vi "Read_Write_Heartbeat_VI.vi"() -> ()   [LabVIEW 2017]
uses:
  b0f9d034-c42f-4ddb-9695-d4b8d01b2041.vi
  <vilib>/Plasmionique/MB Master/MB_Master_TCP/MB_Master_TCP.lvclass
  C:/Program Files (x86)/National Instruments/LabVIEW 2017/vi.lib/Plasmionique/MB Master/MB_Master/MB_Master.lvclass
  <vilib>/Plasmionique/MB Master/MB Master.lvlib
panel:
  out "Heartbeat Value to BMS":i32
  out "BMS IP Address":string
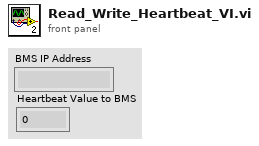
[diagram p1: front panel]
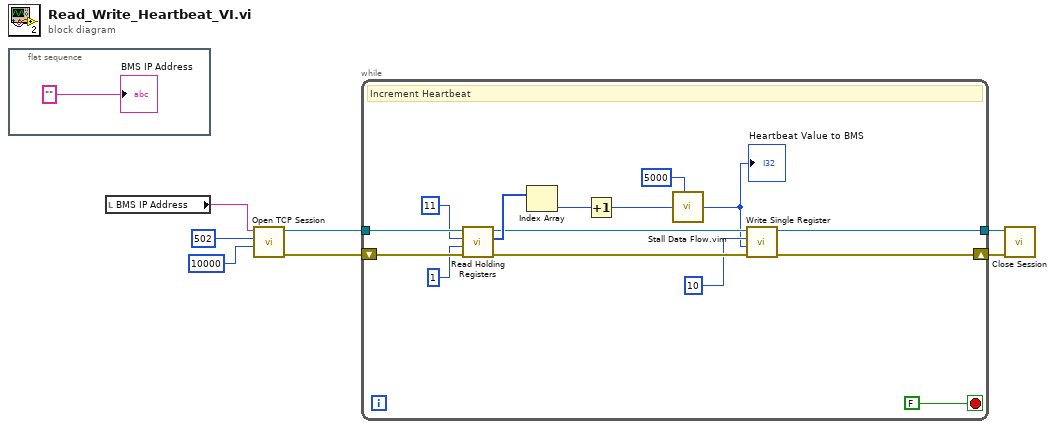
[diagram p0: block diagram]
diagram:
  n1 = flat-sequence {
    frame #0 {
      "BMS IP Address" <- "" ("String")
    }
  }
  n2 = local read "BMS IP Address"() -> (w3:string)
  n3 = call <vilib>:"Open TCP Session.vi"("Timeout (10000)"=10000, "Port (502)"=u16 502, "IP Address"=w3) -> ("error out"=w6:errorcluster, "MB_TCP session"=w7:refnum<class "MB_Master_TCP.lvclass">)  [unwired: 7 in]
  n4 = while {
    tunnel: w7 -> [w22]
    shift-right: [w11] -> w2
    shift-left: w6 -> [w21]
    tunnel: [w10] -> w1
    stop <- FALSE stop-if-true
    # "Increment Heartbeat"
    n5 = call <vilib>:"Read Holding Registers.vi"("error in (no error)"=w21, "quantity"=u16 1, "starting address"=u16 11, "MB session in"=w22) -> ("error out"=w13:errorcluster, "Registers"=w18:u16[], "MB session out"=w14:refnum<class "MB_Master_TCP.lvclass">)  [unwired: 5 in]
    n6 = Index Array(array=w18) -> (element=w17:u16)  [unwired: 1 in]
    n7 = Increment(x=w17) -> (x+1=w16:u16)
    n8 = call "Stall Data Flow.vim"("value in"=w16, "milliseconds to wait"=u32 5000) -> ("value out"=w9:u16)  [unwired: 1 out]
    "Heartbeat Value to BMS" <- w9
    n9 = call <vilib>:"Write Single Register.vi"("error in (no error)"=w13, "value"=w9, "address"=u16 10, "MB session in"=w14) -> ("error out"=w11:errorcluster, "MB session out"=w10:refnum<class "MB_Master_TCP.lvclass">)  [unwired: 6 in]
  }
  n10 = call-dynamic "Close Session.vi"("error in (no error)"=w2, "MB TCP session"=w1) -> ()  [unwired: 9 in, 1 out]
